vi "fpga_ARC ABS Less One (I8).vi"(1 "x [I8]":i8) -> (0 "abs(x)-1":u8)   [LabVIEW 2011, in "NI_EP_Resample_FPGA.lvlib"]
uses:
  <vilib>/addons/Electrical Power/PQ/Resampling/NI_EP_Resample_FPGA.lvlib
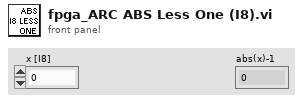
[diagram p1: front panel]
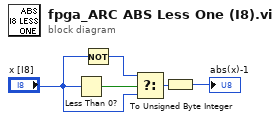
[diagram p0: block diagram]
diagram:
  n1 = Less Than 0?(x="x [I8]") -> (x < 0?=w5:bool)
  n2 = Not(x="x [I8]") -> (.not. x?=w4:i8)
  n3 = Select(t=w4, s=w5, f="x [I8]") -> (s? t:f=w2:i8)
  n4 = To Unsigned Byte Integer(number=w2) -> (unsigned 8bit integer=→"abs(x)-1":u8)
